vi "fpga_LP2 Filter (M Class_60Hz).vi"(0 "input data":fxp<+/-,32,5>[](array[numeric]), 1 "reset":bool, 5 "#Ch":fxp<+,5,5>=16.0, 7 "Memory In":refnum<k21>="coefROM", 9 "input valid":bool) -> (4 "output data":fxp<+/-,32,6>[](array[numeric]), 10 "output valid":bool, 14 "ready for input":bool, 15 "error":i32)   [LabVIEW 2013, in "NI_EP_PMU_FPGA.lvlib"]
doc: "----------------------\n\nThis filter is configured as follows:\n\n<b>Filter Configuration</b>\nType: Single Rate\nStructure: FIR Direct Form\n\n<b>Input Data Type</b>\nType: fixed-point <±,32,5> [-1.600000E+1,1.600000E+1]:7.450581E-9\n\n<b>Output Data Type</b>\nType: fixed-point <±,32,6> [-3.200000E+1,3.200000E+1]:1.490116E-8\nRounding mode: Truncate\nOverflow mode: Wrap\n\n<b>Implementation</b>\nNumber of channels: 16\nMaximum input sampling rate per channel @ 40MHz: 2.104kHz\nGain processing: On Host\nMethod: Multiply-Accumulate\nNumber of multiply pipeline stages: 1\nMultiply register in: False\nNumber of adder levels per register: 2\nState memory: Block Memory\nCoefficient memory: Block Memory\n\n<b>Execution Mode</b>\nInside single-cycle Timed Loop\nThroughput: 1188 cycles/sample\n\n<b>Estimated Resources</b>\nNumber of multiply-accumulate units: 1\nMultiply operation: I32.5 x I16.-6 => I48.6"
uses:
  <vilib>/addons/Electrical Power/PMU/NI_EP_PMU_FPGA.lvlib
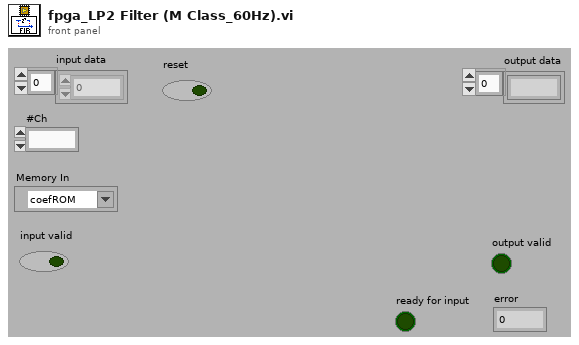
[diagram p1: front panel]
types:
  T1 = cluster{"WREn":bool, "WRAddr":fxp<+,15,15>, "RDAddr":fxp<+,15,15>, "BufWREn":bool, "BufWRAddr":fxp<+,15,15>, "firstRun":bool, "BufFiirstRun":bool}
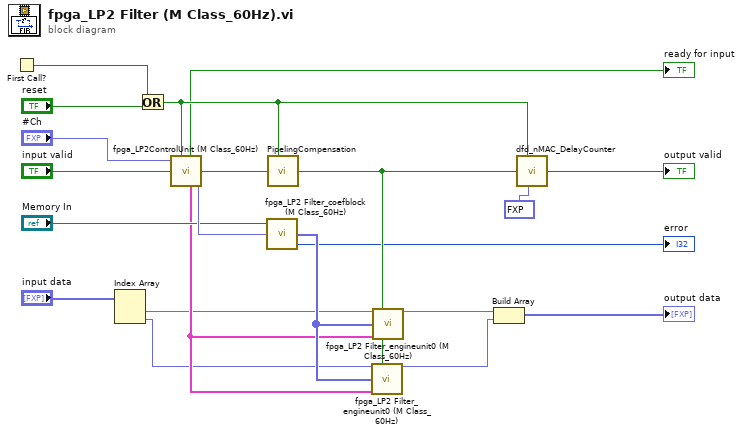
[diagram p0: block diagram]
diagram:
  n1 = First Call?() -> (First Call?: T/F=w18:bool)
  n2 = Index Array(array="input data") -> (element #1=w6:fxp<+/-,32,5>, element #2=w5:fxp<+/-,32,5>)  [unwired: 2 in]
  n3 = Or(x=w18, y="reset") -> (x .or. y?=w17:bool)
  n4 = call <vilib>:"fpga_LP2ControlUnit (M Class_60Hz).vi"("#Ch"="#Ch", "reset"=w17, "input valid"="input valid") -> ("ready for input"=→"ready for input":bool, "output valid"=w20:bool, "opState"=w8:T1, "coefRDAddr"=w15:fxp<+,11,11>)  [unwired: 3 in]
  n5 = call <vilib>:"fpga_LP2 Filter_coefblock (M Class_60Hz).vi"("Memory In"="Memory In", "coefAddr"=w15) -> ("coefficients"=w9:fxp<+/-,19,-3>[], "error"=→"error":i32)  [unwired: 6 in]
  n6 = call "PipelingCompensation"("reset"=w17, "data in"=w20) -> ("data out"=w10:bool)  [unwired: 7 in]
  n7 = call <vilib>:"fpga_LP2 Filter_engineunit0 (M Class_60Hz).vi"("input data"=w5, "ACC_Load"=w10, "coefficients"=w9, "opState"=w8) -> ("output data"=w3:fxp<+/-,32,6>)  [unwired: 11 in]
  n8 = call <vilib>:"fpga_LP2 Filter_engineunit0 (M Class_60Hz).vi"("input data"=w6, "ACC_Load"=w10, "coefficients"=w9, "opState"=w8) -> ("output data"=w4:fxp<+/-,32,6>)  [unwired: 11 in]
  n9 = Build Array(w4, w3) -> (→"output data":fxp<+/-,32,6>[])
  n10 = call "dfd_nMAC_DelayCounter.vi"("reset"=w17, "data in"=w10, "#delay"=fxp<+,11,11> 1188.0 ("#TPPM")) -> ("data out"=→"output valid":bool)  [unwired: 6 in]
